vi "Send Set PID Gains.vi"(8 "error in (no error)":errorcluster, 10 "PID gains":T1, 11 "Message Queue in":refnum<queue>) -> (0 "error out":errorcluster, 3 "Message Queue out":refnum<queue>)   [LabVIEW 2024, in "PID Loop.lvlib" / "Set PID Gains.lvclass"]
uses:
  Set PID Gains.lvclass
  Set PID Gains.lvclass/Set PID Gains.ctl
  C:/Users/uspoaotto/OneDrive - Oregon Tool/Desktop/working copies/helperLoop/src/OOQMH/Message/Message.lvclass
  C:/Users/uspoaotto/OneDrive - Oregon Tool/Desktop/working copies/helperLoop/src/PID Loop/Set PID Gains/Set PID Gains.lvclass
  OOQMH/Message/Message.lvclass
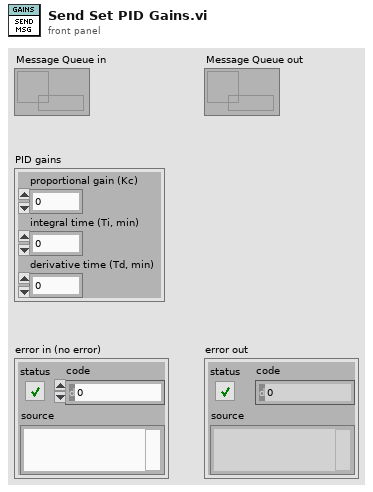
[diagram p1: front panel]
types:
  T1 = cluster{"proportional gain (Kc)":dbl, "integral time (Ti, min)":dbl, "derivative time (Td, min)":dbl}
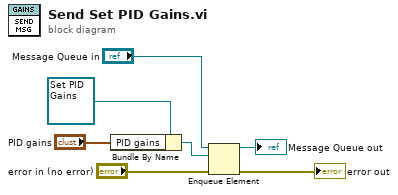
[diagram p0: block diagram]
diagram:
  n1 = Bundle By Name(cluster=refnum<class "Set PID Gains.lvclass"> refnum ("PID Loop.lvlib:Set PID Gains.lvclass"), "PID gains"="PID gains") -> (w3:refnum<class "Set PID Gains.lvclass">)
  n2 = Enqueue Element(queue="Message Queue in", element=w3, error in (no error)="error in (no error)") -> (queue out=→"Message Queue out":refnum<queue>, error out=→"error out":errorcluster)  [unwired: 1 in, 1 out]
